vi "UM.vi"() -> (1 "annulla?":bool, 2 "RingText.Text":string)   [LabVIEW 2019]
panel:
  in  "annulla":bool
  in  "OK Button":bool
  in  "Unità di Misura":T1
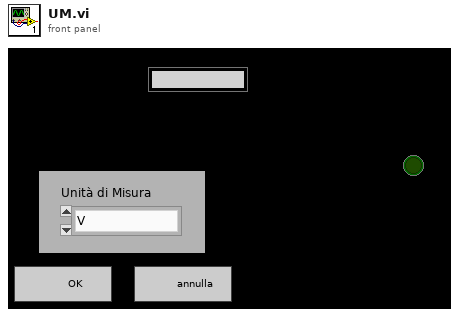
[diagram p1: front panel]
types:
  T1 = typedef "UnitàMisura.ctl" = enum16{"V", "mA", "Bar", "RPM", "m3/s", "m3/min", "m3/h", "l/s", "l/min", "in3/min", "ft3/min", "gpm", "igpm", "igph", "%", "°C", "m", "Nm", "A"}
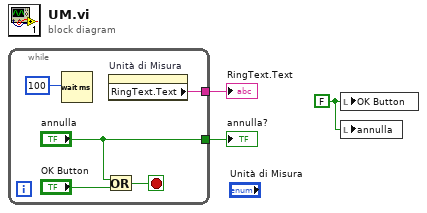
[diagram p0: block diagram]
diagram:
  w2 = FALSE ("OK Button")
  n1 = while {
    tunnel: [w6] -> w3
    tunnel: ["annulla"] -> w1
    stop <- w5 stop-if-true
    n2 = Wait (ms)(milliseconds to wait=u32 100) -> ()  [unwired: 1 out]
    n3 = Or(x="annulla", y="OK Button") -> (x .or. y?=w5:bool)
    n4 = property on="Unità di Misura" class="Enum (strict)"() -> ("RingText.Text"=w6:string)  [unwired: 2 in, 2 out]
  }
  "RingText.Text" <- w3
  "annulla?" <- w1
  n5 = local write "OK Button"(w2) -> ()
  n6 = local write "annulla"(w2) -> ()
